vi "Main v0.3.vi"() -> ()   [LabVIEW 2017]
doc: "This template is for the Queued Message Handler design pattern.\n\nThe Event Handling Loop generates messages based on user interface actions.\n\nThe Message Handling Loop processes messages generated by the Event Handling Loop, or by other messages. The messages are string values, so new messages can be added easily to the Message Cases case structure in the Message Handling Loop. Each message cluster can also provide an optional value for Message Data, which is a variant that can be converted to whatever message-specific data is required."
uses:
  Controls/Main Tabs.ctl
  Controls/Auto.ctl
  RT/Controls/Auto Delays.ctl
  RT/Controls/Auto Times.ctl
  Controls/UI Data.ctl
  support/Message Queue/Enqueue Message (Single).vi
  <vilib>/Utility/error.llb/Error Cluster From Error Code.vi
  <vilib>/ErrorRing/Error Ring.xnode
  support/Message Queue/Message Queue.lvlib
  support/User Event - Stop/User Event - Stop.lvlib
panel:
  out "Date-Time":string caption="Dip-Tube Assembly Automation (HMI) v0.3"
  out "Main Tab":T1
  in  "Autocycle":T2
  in  "Manual":bool
  in  "Parameters":bool
  in  "Maintenance":bool
  in  "Save Para":bool
  in  "Home Para":bool
  in  "ParaTab":T3(tab)
  in  "StopperRearDelay":dbl format="%#.2f"
  in  "StopperFrontDelay":dbl format="%#.2f"
  in  "MaxAlarms":dbl caption="Max Alarms in 1 Minute" format="%#.2f"
  in  "MaxConsecutive":dbl caption="Max Consecutive Alarms" format="%#.2f"
  in  "Gate Close Delay":dbl format="%#.2f"
  in  "Gate Open Delay":dbl format="%#.2f"
  in  "BF Off Delay":dbl format="%#.2f"
  in  "BF On Delay":dbl format="%#.2f"
  in  "DelayAfterReject":dbl format="%#.2f"
  in  "MeasurementTime":dbl format="%#.2f"
  in  "DelayAfterMesFront":dbl format="%#.2f"
  in  "DelayAfterCut":dbl format="%#.2f"
  in  "DelayAfterCutClamp":dbl format="%#.2f"
  in  "DelayAfterInsClamp":dbl format="%#.2f"
  in  "DelayToClose":dbl format="%#.2f"
  in  "DelayToOpen":dbl format="%#.2f"
  in  "DelayAfterInsertion":dbl format="%#.2f"
  in  "DelayBeforeInsertion":dbl format="%#.2f"
  in  "AgitatorUpTime":dbl format="%#.2f"
  in  "AgitatorDownTime":dbl format="%#.2f"
  in  "Enable Reject?":bool
  in  "Enable Measure?":bool
  in  "Enable Index?":bool
  in  "Enable PF?":bool
  in  "Auto Delays":T4={"Agitator Delays"=[1000], "TF Delays"=[1000], "Insertion Delays"=[1000, 1000], "Cutting Delays"=[1000, 1000, 1000], "PF Delays"=[1000], "Measur. Delays"=[1000]}
  in  "Enable Cutting?":bool
  in  "Enable Insertion?":bool
  in  "Run Manual":bool
  in  "Enable TF?":bool
  in  "Home Manual":bool
  out "Status":T6
  out "Measurements":cluster{"1":dbl, "2":dbl, "3":dbl, "4":dbl}
  in  "All IO":bool
  in  "Stats":bool
  in  "Home AC":bool
  out "Status":string
  out "Count":dbl format="%06.0f"
  out "Count 3":dbl caption="Cycle Time" format="%0.2f"
  out "Count 2":dbl caption="Rejects" format="%06.0f"
  in  "Statuses":string[][](table)
  in  "Exit":bool
  # "Vision Harmony Dip-Tube Assembly Automation"
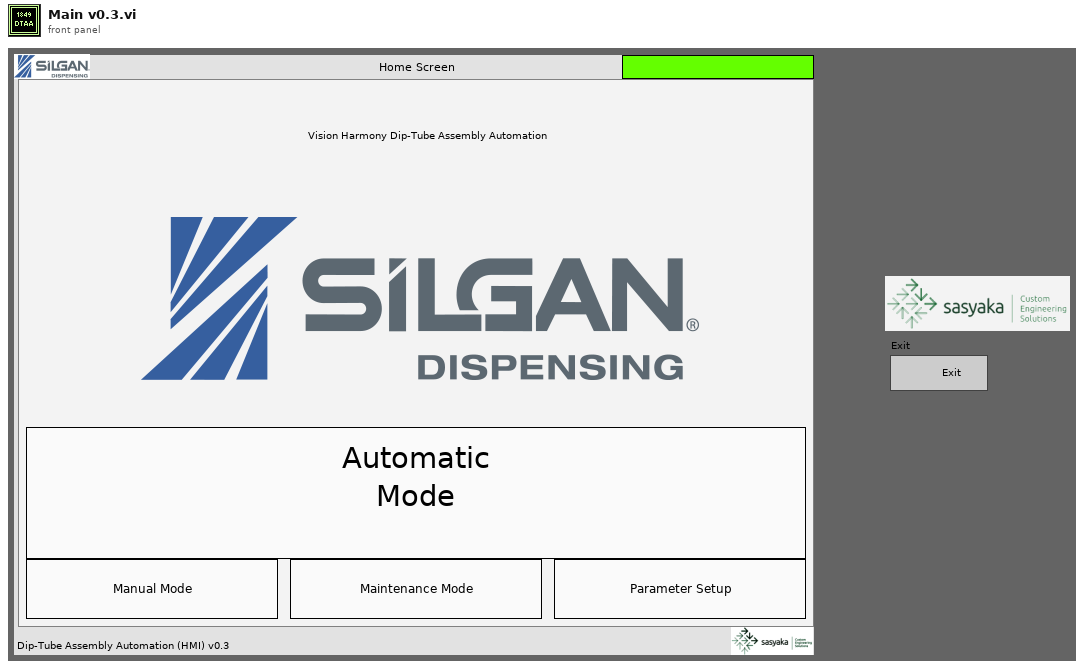
[diagram p1: front panel]
types:
  T1 = typedef "Main Tabs.ctl" = enum32{"Home Screen", "Parameter Setup", "Manual Mode", "Autocycle"}
  T2 = typedef "Auto.ctl" = bool
  T3 = enum32{"General & Indexing", "Bowl Feeder & Pump Conveyor", "Cutting, Measurement & Rejection", "Tube Feeder & Insertion"}
  T4 = typedef "Auto Delays.ctl" = cluster{"Agitator Delays":u32[], "TF Delays":u32[], "Insertion Delays":u32[], "Cutting Delays":u32[], "PF Delays":u32[], "Measur. Delays":u32[]}
  T5 = typedef "Auto Times.ctl" = cluster{"Index Time":u32, "TF Time":u32, "Insertion Time":u32, "Cutting Time":u32, "PF Time":u32, "Meas. Time":u32}
  T6 = cluster{"Auto Times":T5, "error out":errorcluster}
  T7 = typedef "UI Data.ctl" = cluster{"Main Tab":refnum<vi>}
  T8 = typedef "Message Queue.lvlib/All Message Queues.ctl" = cluster{"UI":refnum<queue>}
  T9 = enum8{"Enabled", "Disabled", "Disabled and Grayed Out"}
  T10 = cluster{"Auto Times":T5, "Measurements":cluster{"1":dbl, "2":dbl, "3":dbl, "4":dbl}, "error out":errorcluster}
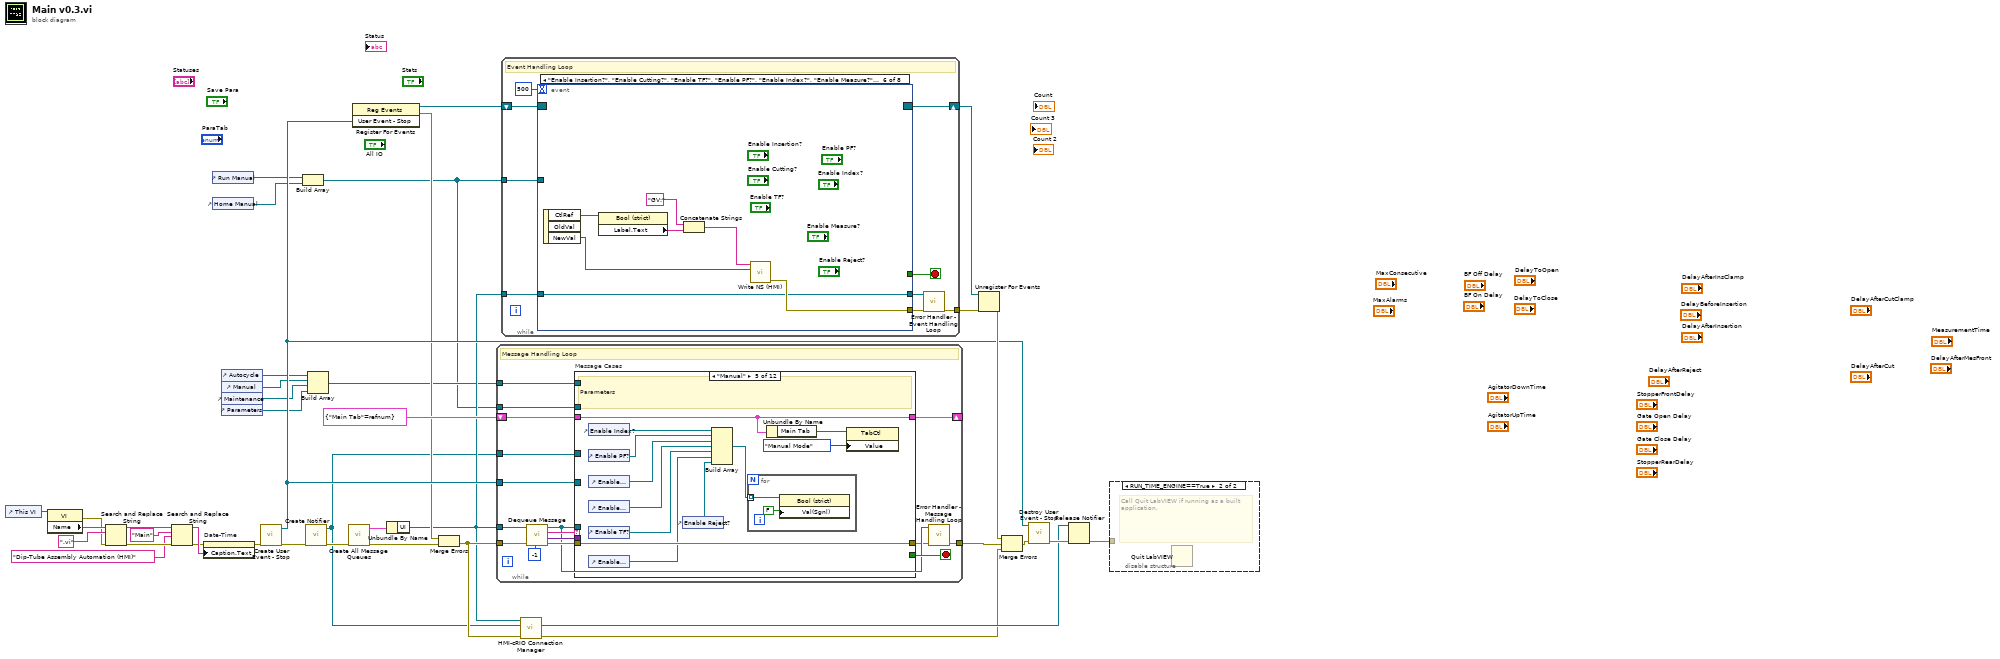
[diagram p0: block diagram]
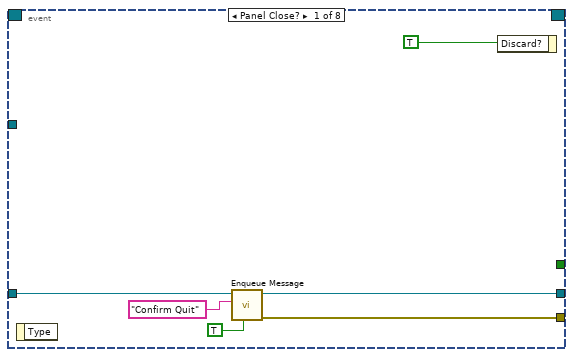
[diagram p2: hidden frame]
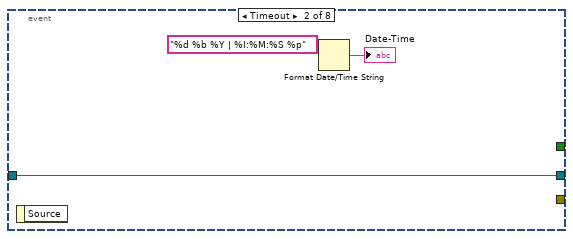
[diagram p3: hidden frame]
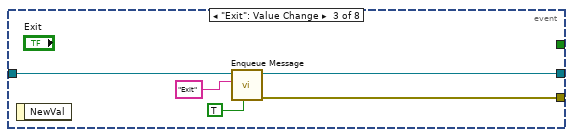
[diagram p4: hidden frame]
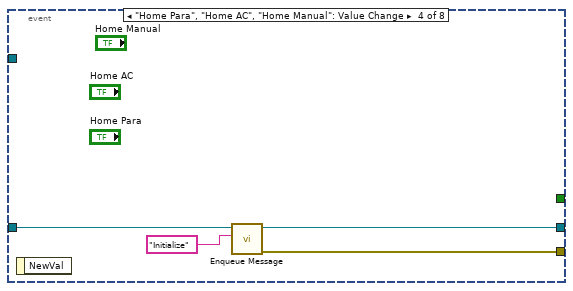
[diagram p5: hidden frame]
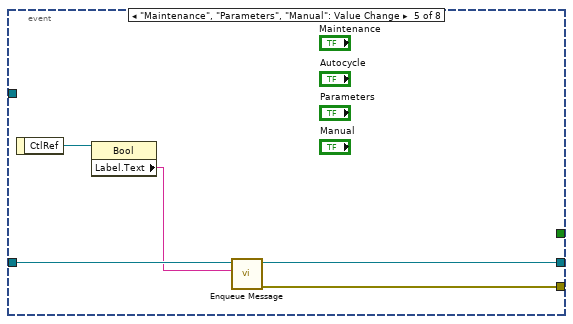
[diagram p6: hidden frame]
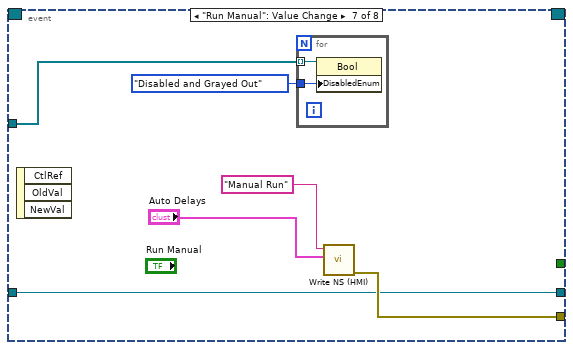
[diagram p7: hidden frame]
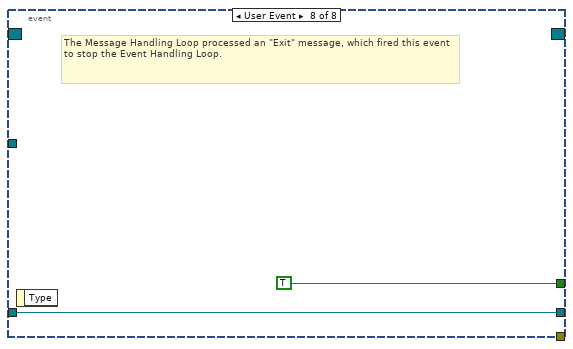
[diagram p8: hidden frame]
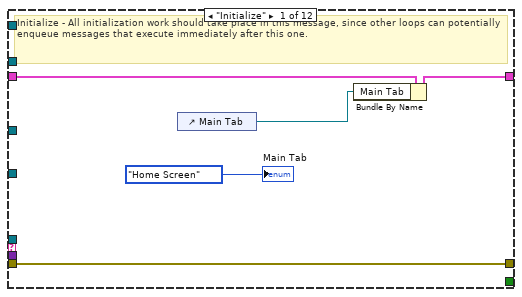
[diagram p9: hidden frame]
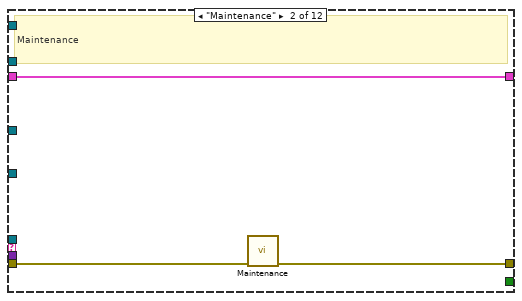
[diagram p10: hidden frame]
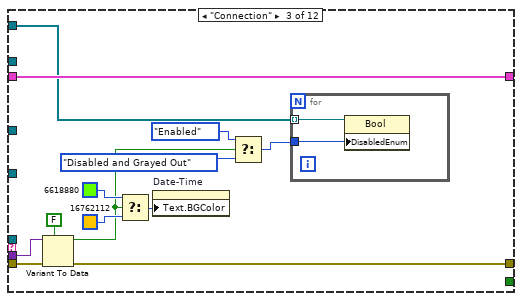
[diagram p11: hidden frame]
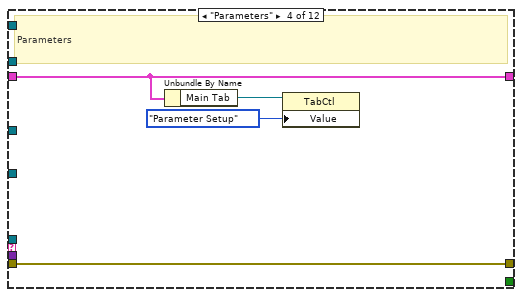
[diagram p12: hidden frame]
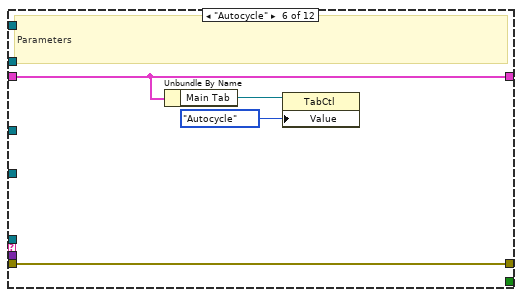
[diagram p13: hidden frame]
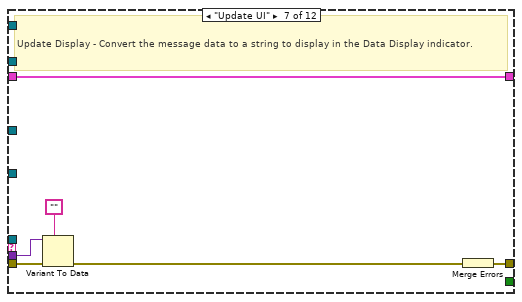
[diagram p14: hidden frame]
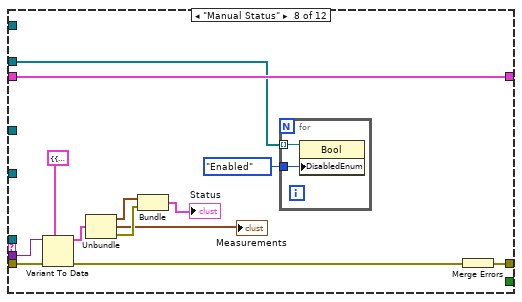
[diagram p15: hidden frame]
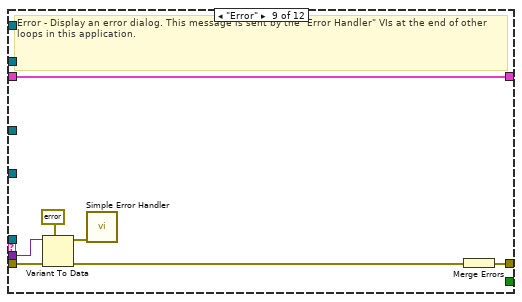
[diagram p16: hidden frame]
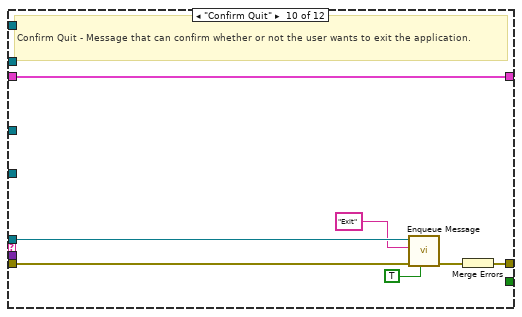
[diagram p17: hidden frame]
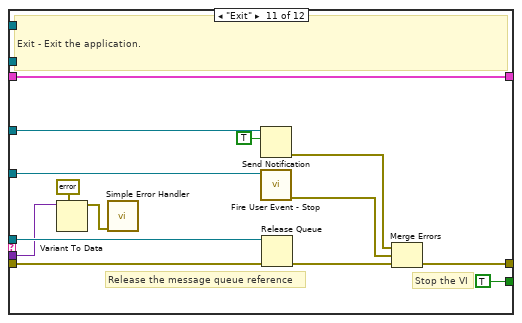
[diagram p18: hidden frame]
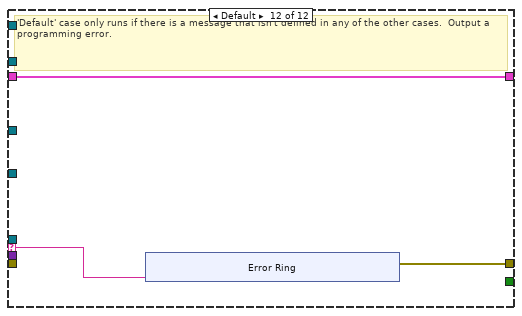
[diagram p19: hidden frame]
diagram:
  n1 = control-ref of="This VI"() -> (w8:refnum<vi>)
  n2 = property class="VI"(reference=w8) -> (error out=w7:errorcluster, "Name"=w14:string)  [unwired: 1 in, 1 out]
  n3 = Search and Replace String(input string=w14, search string=".vi", error in=w7) -> (result string=w12:string, error out=w11:errorcluster)  [unwired: 5 in, 2 out]
  n4 = Search and Replace String(input string=w12, search string="Main", replace string="Dip-Tube Assembly Automation (HMI)" ("replace string (\"\")"), error in=w11) -> (result string=w6:string, error out=w5:errorcluster)  [unwired: 4 in, 2 out]
  n5 = property on="Date-Time" class="Str"(error in=w5, "Caption.Text"=w6) -> (error out=w4:errorcluster)  [unwired: 1 in, 1 out]
  n6 = control-ref of="Run Manual"() -> (w3:refnum<vi>)
  n7 = control-ref of="Home Manual"() -> (w2:refnum<vi>)
  n8 = control-ref of="Autocycle"() -> (w19:refnum<vi>)
  n9 = control-ref of="Manual"() -> (w18:refnum<vi>)
  n10 = control-ref of="Maintenance"() -> (w17:refnum<vi>)
  n11 = control-ref of="Parameters"() -> (w16:refnum<vi>)
  n12 = call "Create User Event - Stop.vi"("error in (no error)"=w4) -> ("error out"=w26:errorcluster, "User Event - Stop"=w30:refnum<user-event>)  [unwired: 9 in]
  n13 = Build Array(w3, w2) -> (w1:refnum<vi>[])
  n14 = call "Create Notifier.vi"("error in (no error)"=w26) -> ("error out"=w25:errorcluster, "notifier out"=w20:refnum<notifier>)  [unwired: 9 in]
  n15 = Build Array(w19, w18, w17, w16) -> (w15:refnum<vi>[])
  n16 = call "Create All Message Queues.vi"("error in (no error)"=w25) -> ("error out"=w39:errorcluster, "Message Queues out"=w38:T8)  [unwired: 9 in]
  n17 = register-events(w30) -> (reference out=w31:refnum<event-registration>, error out=w29:errorcluster)  [unwired: 2 in]
  n18 = Unbundle By Name(w38) -> ("UI"=w27:refnum<queue>)
  n19 = Merge Errors(w29, w39) -> (w28:errorcluster)
  n20 = while {
    tunnel: w27 -> [w47]
    shift-right: [w54] -> _
    shift-left: T7 {"Main Tab"=refnum} ("Data Cluster") -> [w55]
    tunnel: w30 -> [w52]
    tunnel: w28 -> [w51]
    tunnel: [w45] -> w37
    tunnel: w20 -> [w42]
    tunnel: w15 -> [w41]
    tunnel: w1 -> [w40]
    stop <- w53 stop-if-true
    # "Message Handling Loop"
    n21 = call "Dequeue Message.vi"("timeout"=-1, "error in (no error)"=w51, "Message Queue"=w47) -> ("error out"=w50:errorcluster, "Message Data"=w48:variant, "Message"=w49:string, "dup Message Queue"=w46:refnum<queue>)  [unwired: 5 in]
    n22 = case "Message Cases" shown="\"Manual\"" w49 {
      selector: w49 -> [_ _ _ _ _ _ _ _ _ _ _ w150]
      tunnel: w46 -> [_ _ _ _ _ _ _ _ _ w131 w149 _]
      tunnel: w50 -> [w60 w62 w74 w82 w94 w100 w104 w117 w128 w135 w142 _]
      tunnel: [w60 w61 w73 w82 w94 w100 w105 w118 w122 w133 w145 w151] -> w44
      tunnel: w55 -> [w59 w63 w76 w81 w93 w99 w106 w119 w127 w134 w148 w152]
      tunnel: [w58 w63 w76 w81 w93 w99 w106 w119 w127 w134 w148 w152] -> w54
      tunnel: [_ _ _ _ _ _ _ _ _ _ TRUE _] -> w53
      tunnel: w48 -> [_ _ w72 _ _ _ w103 w116 w126 _ w139 _]
      tunnel: w52 -> [_ _ _ _ _ _ _ _ _ _ w144 _]
      tunnel: w42 -> [_ _ _ _ _ _ _ _ _ _ w138 _]
      tunnel: w41 -> [_ _ w68 _ _ _ _ _ _ _ _ _]
      tunnel: w40 -> [_ _ _ _ _ _ _ w113 _ _ _ _]
      frame "Initialize" {
        # "Initialize - All initialization work should take place in this message, since other loops can potentially enqueue messages that execute immediately after this one."
        n23 = control-ref of="Main Tab"() -> (w57:refnum<vi>)
        n24 = Bundle By Name(cluster=w59, "Main Tab"=w57) -> (w58:T7)
        "Main Tab" <- Main_Tabs."Home Screen" ("Main Tab")
      }
      frame "Maintenance" {
        # "Maintenance"
        n25 = call "Maintenance.vi"("Error In"=w62) -> ("Error out"=w61:errorcluster)  [unwired: 10 in]
      }
      frame "Connection" {
        n26 = Variant To Data(error in=w74, type=FALSE, Variant=w72) -> (data=w67:bool, error out=w73:errorcluster)
        n27 = Select(t=u32 6618880 ("Text.Text Colors:BG Color"), s=w67, f=u32 16762112 ("Text.Text Colors:BG Color")) -> (s? t:f=w69:u32)
        n28 = property on="Date-Time" class="Str"("Text.BGColor"=w69) -> ()  [unwired: 2 in, 2 out]
        n29 = Select(t=T9."Enabled" ("Disabled"), s=w67, f=T9."Disabled and Grayed Out") -> (s? t:f=w65:T9)
        n30 = for {
          tunnel: w68 -> [w78] mode=indexing
          tunnel: w65 -> [w77]
          n31 = property class="Bool"(reference=w78, "DisabledEnum"=w77) -> ()  [unwired: 1 in, 2 out]
        }
      }
      frame "Parameters" {
        # "Parameters"
        n32 = Unbundle By Name(w81) -> ("Main Tab"=w80:refnum<vi>)
        n33 = property class="TabCtl"(reference=w80, "Value"=Main_Tabs."Parameter Setup" ("Main Tab")) -> ()  [unwired: 1 in, 2 out]
      }
      frame "Manual" {
        # "Parameters"
        n34 = control-ref of="Enable Index?"() -> (w90:refnum<vi>)
        n35 = control-ref of="Enable PF?"() -> (w89:refnum<vi>)
        n36 = control-ref of="Enable Cutting?"() -> (w88:refnum<vi>)
        n37 = control-ref of="Enable Insertion?"() -> (w87:refnum<vi>)
        n38 = control-ref of="Enable TF?"() -> (w86:refnum<vi>)
        n39 = control-ref of="Enable Measure?"() -> (w84:refnum<vi>)
        n40 = control-ref of="Enable Reject?"() -> (w83:refnum<vi>)
        n41 = Build Array(w90, w89, w88, w87, w86, w84, w83) -> (w85:refnum<vi>[])
        n42 = for {
          tunnel: w85 -> [w96] mode=indexing
          n43 = property class="Bool (strict)"(reference=w96, "Val(Sgnl)"=FALSE ("Value (Signaling)")) -> ()  [unwired: 1 in, 2 out]
        }
        n44 = Unbundle By Name(w93) -> ("Main Tab"=w92:refnum<vi>)
        n45 = property class="TabCtl"(reference=w92, "Value"=Main_Tabs."Manual Mode" ("Main Tab")) -> ()  [unwired: 1 in, 2 out]
      }
      frame "Autocycle" {
        # "Parameters"
        n46 = Unbundle By Name(w99) -> ("Main Tab"=w98:refnum<vi>)
        n47 = property class="TabCtl"(reference=w98, "Value"=Main_Tabs."Autocycle" ("Main Tab")) -> ()  [unwired: 1 in, 2 out]
      }
      frame "Update UI" {
        # "Update Display - Convert the message data to a string to display in the Data Display indicator."
        n48 = Variant To Data(error in=w104, type="", Variant=w103) -> (error out=w101:errorcluster)  [unwired: 1 out]
        n49 = Merge Errors(w101) -> (w105:errorcluster)
      }
      frame "Manual Status" {
        n50 = Variant To Data(error in=w117, type=T10 {"Auto Times"={"Index Time"=0, "TF Time"=0, "Insertion Time"=0, "Cutting Time"=0, "PF Time"=0, "Meas. Time"=0}, "Measurements"={"1"=0.0, "2"=0.0, "3"=0.0, "4"=0.0}, "error out"={"status"=FALSE, "code"=0, "source"=""}} ("cluster"), Variant=w116) -> (data=w111:T10, error out=w115:errorcluster)
        n51 = Unbundle(w111) -> ("Auto Times"=w110:T5, "Measurements"=→"Measurements":cluster{"1":dbl, "2":dbl, "3":dbl, "4":dbl}, "error out"=w109:errorcluster)
        n52 = Bundle("Auto Times"=w110, "error out"=w109) -> (→"Status":T6)  [unwired: 1 in]
        n53 = for {
          tunnel: w113 -> [w121] mode=indexing
          tunnel: T9."Enabled" ("Disabled") -> [w120]
          n54 = property class="Bool"(reference=w121, "DisabledEnum"=w120) -> ()  [unwired: 1 in, 2 out]
        }
        n55 = Merge Errors(w115) -> (w118:errorcluster)
      }
      frame "Error" {
        # "Error - Display an error dialog. This message is sent by the \"Error Handler\" VIs at the end of other loops in this application."
        n56 = Variant To Data(error in=w128, type=errorcluster {"status"=FALSE, "code"=0, "source"=""} ("error constant"), Variant=w126) -> (data=w124:errorcluster, error out=w123:errorcluster)
        n57 = call <vilib>:"Simple Error Handler.vi"("error in (no error)"=w124) -> ()  [unwired: 4 in, 5 out]
        n58 = Merge Errors(w123) -> (w122:errorcluster)
      }
      frame "Confirm Quit" {
        # "Confirm Quit - Message that can confirm whether or not the user wants to exit the application."
        n59 = call-poly "Enqueue Message.vi"("Priority Message? (F)"=TRUE, "error in (no error)"=w135, "Message"="Exit", "Message Queue"=w131) -> ("error out"=w132:errorcluster)  [unwired: 6 in, 1 out]
        n60 = Merge Errors(w132) -> (w133:errorcluster)
      }
      frame "Exit" {
        # "Stop the VI"
        # "Release the message queue reference"
        # "Exit - Exit the application."
        n61 = Variant To Data(type=errorcluster {"status"=FALSE, "code"=0, "source"=""} ("error constant"), Variant=w139) -> (data=w140:errorcluster)  [unwired: 1 in, 1 out]
        n62 = call <vilib>:"Simple Error Handler.vi"("error in (no error)"=w140) -> ()  [unwired: 4 in, 5 out]
        n63 = Send Notification(notification=TRUE, notifier=w138) -> (error out=w136:errorcluster)  [unwired: 1 in, 1 out]
        n64 = call "Fire User Event - Stop.vi"("User Event - Stop"=w144) -> ("error out"=w143:errorcluster)  [unwired: 10 in]
        n65 = Release Queue(queue=w149, error in (no error)=w142) -> (error out=w146:errorcluster)  [unwired: 1 in, 2 out]
        n66 = Merge Errors(w136, w143, w146) -> (w145:errorcluster)
      }
      frame Default {
        # "'Default' case only runs if there is a message that isn't defined in any of the other cases.  Output a programming error."
        n67 = xnode "Error Ring"("parameter 0"=w150) -> ("error out"=w151:errorcluster)
      }
    }
    n68 = call "Error Handler - Message Handling Loop.vi"("error in (no error)"=w44, "Message Queue"=w46) -> ("dup error in"=w45:errorcluster)  [unwired: 8 in, 1 out]
  }
  n69 = while {
    tunnel: w27 -> [w168]
    shift-right: [w166] -> w34
    shift-left: w31 -> [w167]
    tunnel: [w162] -> w32
    tunnel: w1 -> [w160]
    stop <- w164 stop-if-true
    # "Event Handling Loop"
    n70 = event shown="[5] \"Enable Insertion?\", \"Enable Cutting?\", \"Enable TF?\", \"Enable PF?\", \"Enable Index?\", \"Enable Measure?\", \"Enable Reject?\": Value Change" {
      selector: w167 -> [_ _ _ _ _ _ _ _]
      dyn-events: [_ _ _ _ _ _ _ _] -> w166
      timeout: 500 -> [_ _ _ _ _ _ _ _]
      tunnel: [_ _ _ _ _ _ _ TRUE ("Discard?")] -> w164
      tunnel: w168 -> [w173 w177 w182 w186 w191 w196 w203 w208]
      tunnel: [w172 _ w181 w185 w190 w197 w204 _] -> w165
      tunnel: [w171 w177 w180 w184 w189 w196 w203 w208] -> w163
      tunnel: w160 -> [_ _ _ _ _ _ w200 _]
      event Panel Close? {
        n71 = event-data() -> ()  [unwired: 1 in, 1 out]
        n72 = call-poly "Enqueue Message.vi"("Priority Message? (F)"=TRUE, "Message"="Confirm Quit", "Message Queue"=w173) -> ("error out"=w172:errorcluster, "dup Message Queue"=w171:refnum<queue>)  [unwired: 7 in]
        n73 = event-data("Discard?"=TRUE) -> ()  [unwired: 1 in, 1 out]
      }
      event Timeout {
        n74 = event-data() -> ()  [unwired: 1 in, 1 out]
        n75 = Format Date/Time String(time format string (%c)="%d %b %Y | %I:%M:%S %p") -> (date/time string=→"Date-Time":string)  [unwired: 2 in]
      }
      event "Exit": Value Change {
        n76 = event-data() -> ()  [unwired: 1 in, 1 out]
        n77 = call-poly "Enqueue Message.vi"("Priority Message? (F)"=TRUE, "Message"="Exit", "Message Queue"=w182) -> ("error out"=w181:errorcluster, "dup Message Queue"=w180:refnum<queue>)  [unwired: 7 in]
      }
      event "Home Para", "Home AC", "Home Manual": Value Change {
        n78 = event-data() -> ()  [unwired: 1 in, 1 out]
        n79 = call-poly "Enqueue Message.vi"("Message"="Initialize", "Message Queue"=w186) -> ("error out"=w185:errorcluster, "dup Message Queue"=w184:refnum<queue>)  [unwired: 8 in]
      }
      event "Maintenance", "Parameters", "Manual": Value Change {
        n80 = event-data() -> ("CtlRef"=w188:refnum<vi>)  [unwired: 1 in]
        n81 = property class="Bool"(reference=w188) -> ("Label.Text"=w187:string)  [unwired: 1 in, 2 out]
        n82 = call-poly "Enqueue Message.vi"("Message"=w187, "Message Queue"=w191) -> ("error out"=w190:errorcluster, "dup Message Queue"=w189:refnum<queue>)  [unwired: 8 in]
      }
      event "Enable Insertion?", "Enable Cutting?", "Enable TF?", "Enable PF?", "Enable Index?", "Enable Measure?", "Enable Reject?": Value Change {
        n83 = event-data() -> ("CtlRef"=w198:refnum<vi>, "NewVal"=w192:bool)  [unwired: 1 in, 1 out]
        n84 = property class="Bool (strict)"(reference=w198) -> ("Label.Text"=w195:string)  [unwired: 1 in, 2 out]
        n85 = Concatenate Strings("GV:" ("string"), w195) -> (w193:string)
        n86 = call "Write NS (HMI).vi"("Message Data"=w192, "Message"=w193) -> ("error out"=w197:errorcluster)  [unwired: 9 in]
      }
      event "Run Manual": Value Change {
        n87 = event-data() -> ()  [unwired: 1 in, 3 out]
        n88 = for {
          tunnel: w200 -> [w206] mode=indexing
          tunnel: T9."Disabled and Grayed Out" ("Disabled") -> [w205]
          n89 = property class="Bool"(reference=w206, "DisabledEnum"=w205) -> ()  [unwired: 1 in, 2 out]
        }
        n90 = call "Write NS (HMI).vi"("Message Data"="Auto Delays", "Message"="Manual Run") -> ("error out"=w204:errorcluster)  [unwired: 9 in]
      }
      event User Event {
        # "The Message Handling Loop processed an \"Exit\" message, which fired this event to stop the Event Handling Loop."
        n91 = event-data() -> ()  [unwired: 1 in, 1 out]
      }
    }
    n92 = call "Error Handler - Event Handling Loop.vi"("error in (no error)"=w165, "Message Queue"=w163) -> ("dup error in"=w162:errorcluster)  [unwired: 8 in, 1 out]
  }
  n93 = call "HMI-cRIO Connection Manager.vi"("error in"=w28, "notifier in"=w20, "Queue in"=w27) -> ("error out"=w21:errorcluster, "Notifier out"=w22:refnum<notifier>)  [unwired: 7 in]
  n94 = Unregister For Events(event registration refnum=w34, error in=w32) -> (error out=w35:errorcluster)
  n95 = Merge Errors(w35, w37, w21) -> (w36:errorcluster)
  n96 = call "Destroy User Event - Stop.vi"("error in (no error)"=w36, "User Event - Stop"=w30) -> ("error out"=w24:errorcluster)  [unwired: 9 in]
  n97 = Release Notifier(notifier=w22, error in (no error)=w24) -> (error out=w23:errorcluster)  [unwired: 1 in, 2 out]
  n98 = disable-structure shown="RUN_TIME_ENGINE==True" {
    disable-tunnel: w23 -> [_ _]
    frame condition #0 (active) {
    }
    frame condition #1 {
      # "Call Quit LabVIEW if running as a built application."
      n99 = Quit LabVIEW() -> ()  [unwired: 1 in]
    }
  }
